vi "Fetch IQ vs Slot Measurement Overall Frequency Error.vi"(8 "error in (no error)":errorcluster, 9 "Instance (1)":i32=1 format="%.0g", 11 "VISA resource name":refnum<visa-resource-name>) -> (0 "error out":errorcluster, 1 "Results":dbl[](array[numeric]) format="%.2p", 2 "Reliability":i32, 3 "VISA resource name out":refnum<visa-resource-name>)   [LabVIEW 2020, in "Rohde&Schwarz CMXP GPRF.lvlib"]
doc: "Returns the overall frequency errors.\n\nAttribute:\nRSCMXPGPRF_ATTR_FETCH_IQ_VS_SLOT_MEASUREMENT_OVERALL_FREQUENCY_ERROR\n\nRemote-control command:\nFETCh:GPRF:MEAS<i>:IQVSlot:OFERror?"
uses:
  <instrlib>/Rohde&Schwarz CMXP GPRF/Rohde&Schwarz CMXP GPRF.lvlib
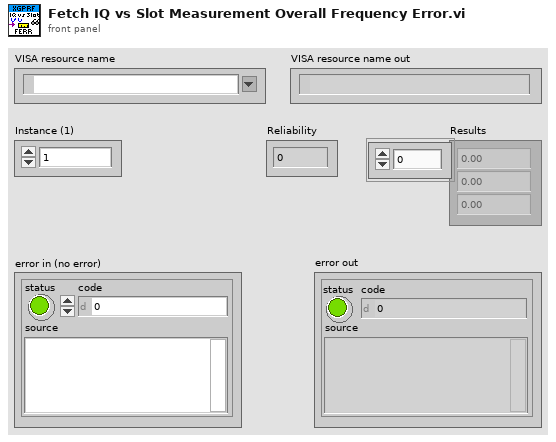
[diagram p1: front panel]
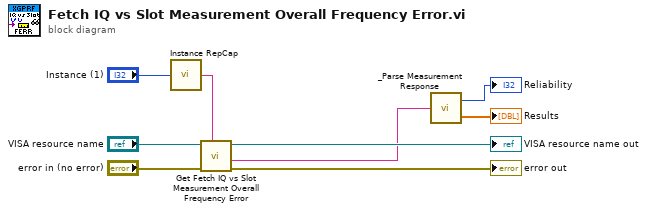
[diagram p0: block diagram]
diagram:
  n1 = call <instrlib>:"Instance RepCap.vi"("Instance in"="Instance (1)") -> ("Instance out"=w9:string)
  n2 = call "Get Fetch IQ vs Slot Measurement Overall Frequency Error"("Repeated Capabilities"=w9, "error in (no error)"="error in (no error)", "instrument handle"="VISA resource name") -> ("error out"=→"error out":errorcluster, "Fetch IQ vs Slot Measurement Overall Frequency Error"=w1:string, "instrument handle out"=→"VISA resource name out":refnum<visa-resource-name>)  [unwired: 6 in]
  n3 = call <instrlib>:"_Parse Measurement Response.vi"("String In"=w1) -> ("Reliability"=→"Reliability":i32, "Data"=→"Results":dbl[])
